vi "test_cRIO daqmx Temp MSS.vi"() -> ()   [LabVIEW 2023]
uses:
  Measure and Stimulus Subsystems/Measure and Stimulus Subsystems.lvclass
  Thermometer/Thermometer DAQmx Base CFG/Thermometer DAQmx Base CFG.lvclass
  Thermometer/Virtual Thermometers/Virt Temperature Reader/Virt Temperature Reader.lvclass
panel:
  out "Temperature Chart":dbl(graph)
  out "Error Out":errorcluster
  in  "Stop":bool
  out "Iteration":i32
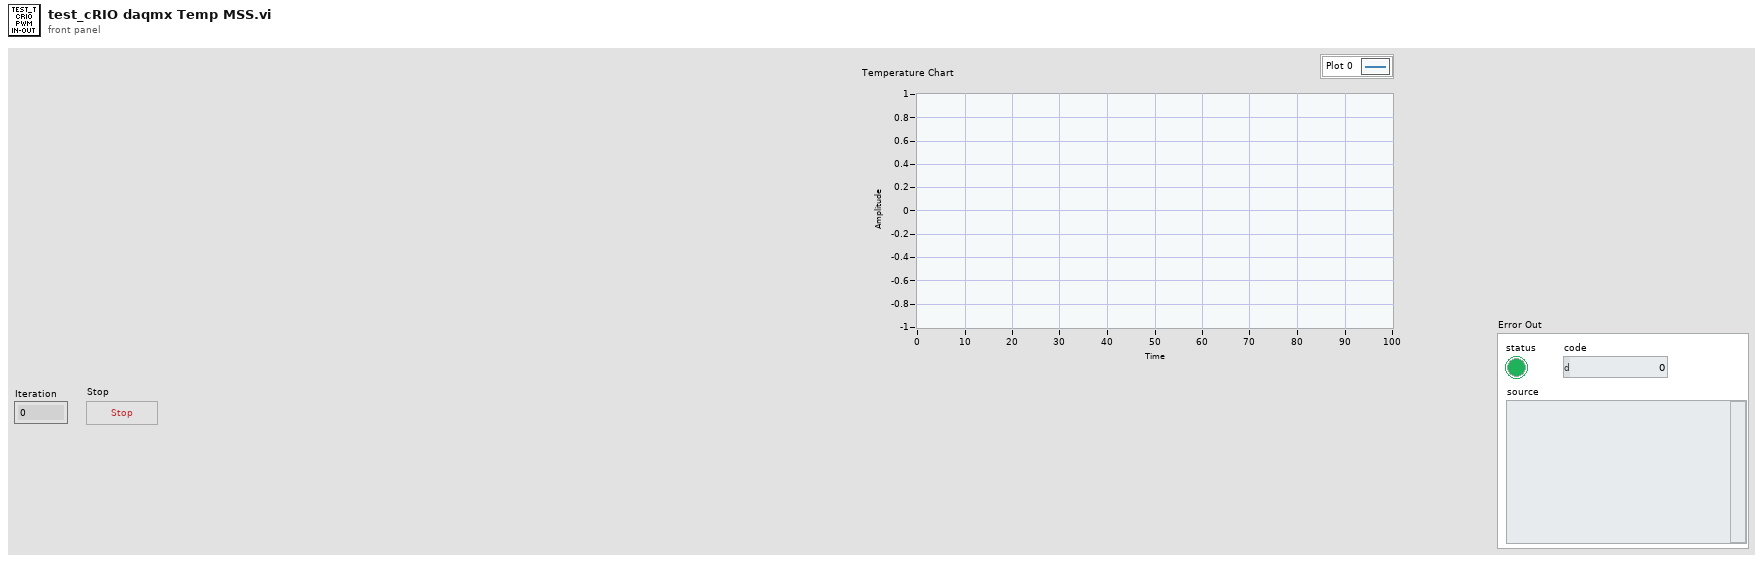
[diagram p1: front panel]
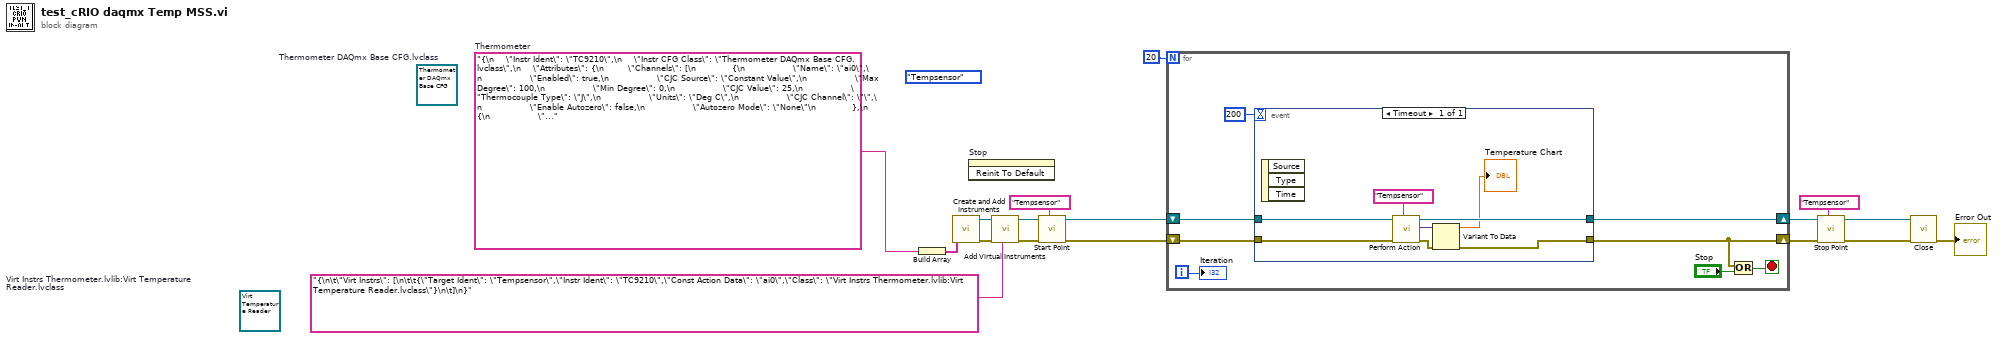
[diagram p0: block diagram]
diagram:
  (unwired) enum16{"Tempsensor"}."Tempsensor"
  (unwired) refnum<class "Virt Temperature Reader.lvclass"> refnum  # Virt Instrs Thermometer.lvlib:Virt Temperature Reader.lvclass
  (unwired) refnum<class "Thermometer DAQmx Base CFG.lvclass"> refnum  # Thermometer DAQmx Base CFG.lvclass
  w9 = "{\n    \"Instr Ident\": \"TC9210\",\n    \"Instr CFG Class\": \"Thermometer DAQmx Base CFG.lvclass\",\n    \"Attributes\": {\n        \"Channels\": [\n            {\n                \"Name\": \"ai0\",\n                \"Enabled\": true,\n                \"CJC Source\": \"Constant Value\",\n                \"Max Degree\": 100,\n                \"Min Degree\": 0,\n                \"CJC Value\": 25,\n                \"Thermocouple Type\": \"J\",\n                \"Units\": \"Deg C\",\n                \"CJC Channel\": \"\",\n                \"Enable Autozero\": false,\n                \"Autozero Mode\": \"None\"\n            },\n            {\n                \"Name\": \"ai1\",\n                \"Enabled\": false,\n                \"CJC Source\": \"Constant Value\",\n                \"Max Degree\": 100,\n                \"Min Degree\": 0,\n                \"CJC Value\": 25,\n                \"Thermocouple Type\": \"J\",\n                \"Units\": \"Deg C\",\n                \"CJC Channel\": \"\",\n                \"Enable Autozero\": false,\n                \"Autozero Mode\": \"None\"\n            },\n            {\n                \"Name\": \"ai2\",\n                \"Enabled\": false,\n                \"CJC Source\": \"Constant Value\",\n                \"Max Degree\": 100,\n                \"Min Degree\": 0,\n                \"CJC Value\": 25,\n                \"Thermocouple Type\": \"J\",\n                \"Units\": \"Deg C\",\n                \"CJC Channel\": \"\",\n                \"Enable Autozero\": false,\n                \"Autozero Mode\": \"None\"\n            },\n            {\n                \"Name\": \"ai3\",\n                \"Enabled\": false,\n                \"CJC Source\": \"Constant Value\",\n                \"Max Degree\": 100,\n                \"Min Degree\": 0,\n                \"CJC Value\": 25,\n                \"Thermocouple Type\": \"J\",\n                \"Units\": \"Deg C\",\n                \"CJC Channel\": \"\",\n                \"Enable Autozero\": false,\n                \"Autozero Mode\": \"None\"\n            }\n        ],\n        \"Timing\": {\n            \"Samples per Channel\": 1000,\n            \"Sample Mode\": \"Continuous Samples\",\n            \"Sample Rate\": 14,\n            \"Sample Clock Source\": \"OnboardClock\",\n            \"Active Edge\": \"Rising\"\n        },\n        \"Trigger\": {\n            \"Trigger Type\": \"No Trigger\"\n        },\n        \"Acquisition\": {\n            \"Relative To\": \"Current Read Position\",\n            \"Overwrite\": \"Do Not Overwrite Unread Samples\",\n            \"Samples per Fetch\": -1,\n            \"Timeout\": 1\n        }\n    }\n}"  # Thermometer
  n1 = Build Array(w9) -> (w8:string[])
  n2 = call "Create and Add Instruments.vi"("Physical Intr CFGs"=w8) -> ("Error Out"=w17:errorcluster, "MSS out"=w4:refnum<class "Measure and Stimulus Subsystems.lvclass">)  [unwired: 9 in]
  n3 = invoke on="Stop" class="Bool (strict)" method="Reinit To Default"() -> ()  [unwired: 3 in, 3 out]
  n4 = call "Add Virtual Instruments.vi"(6:"{\n\t\"Virt Instrs\": [\n\t\t{\"Target Ident\": \"Tempsensor\",\"Instr Ident\": \"TC9210\",\"Const Action Data\": \"ai0\",\"Class\": \"Virt Instrs Thermometer.lvlib:Virt Temperature Reader.lvclass\"}\n\t]\n}", "error in"=w17, "MSS in"=w4) -> ("error out"=w6:errorcluster, "MSS out"=w5:refnum<class "Measure and Stimulus Subsystems.lvclass">)  [unwired: 7 in]
  n5 = call "Start Point.vi"("Point Ident"="Tempsensor" ("Target Identifier"), "error in"=w6, "MSS in"=w5) -> ("error out"=w11:errorcluster, "MSS out"=w7:refnum<class "Measure and Stimulus Subsystems.lvclass">)  [unwired: 7 in]
  n6 = for {
    N: 20 -> [_]
    shift-right: [w20] -> w13
    shift-left: w11 -> [w25]
    shift-right: [w19] -> w15
    shift-left: w7 -> [w21]
    i -> [w22]
    stop <- w23 stop-if-true
    n7 = event shown="[0] Timeout" {
      selector: _ -> [_]
      dyn-events: _ -> [_]
      timeout: 200 -> [_]
      tunnel: w25 -> [w32]
      tunnel: w21 -> [w31]
      tunnel: [w28] -> w20
      tunnel: [w29] -> w19
      event Timeout {
        n8 = event-data() -> ()  [unwired: 1 in, 3 out]
        n9 = call "Perform Action.vi"("Point Ident"="Tempsensor" ("Target Identifier"), "error in"=w32, "MSS in"=w31) -> ("error out"=w30:errorcluster, "Output"=w26:variant, "MSS out"=w29:refnum<class "Measure and Stimulus Subsystems.lvclass">)  [unwired: 6 in]
        n10 = Variant To Data(error in=w30, Variant=w26) -> (data=→"Temperature Chart":dbl, error out=w28:errorcluster)  [unwired: 1 in]
      }
    }
    n11 = Or(x=w20, y="Stop") -> (x .or. y?=w23:bool)
    "Iteration" <- w22
  }
  n12 = call "Stop Point.vi"("Point Ident"="Tempsensor" ("Target Identifier"), "error in"=w13, "MSS in"=w15) -> ("error out"=w16:errorcluster, "MSS out"=w2:refnum<class "Measure and Stimulus Subsystems.lvclass">)  [unwired: 7 in]
  n13 = call "Close.vi"("error in"=w16, "MSS in"=w2) -> ("error out"=→"Error Out":errorcluster)  [unwired: 8 in, 1 out]
